vi "Test Tag For New Test Method Correct When dot in Test name.vi"(8 "error in (no error)":errorcluster, 11 "Result Model Tests in":refnum<class "Result Model Test Enumeration.lvclass">) -> (0 "error out":errorcluster, 3 "Result Model Tests out":refnum<class "Result Model Test Enumeration.lvclass">)   [LabVIEW 2020, in "Result Model Test Enumeration.lvclass"]
uses:
  Result Model Test Enumeration.lvclass
  source/User Interface/Result Model/Result Model.lvclass
  206db1ee-aa99-40b9-8881-171f2a77c34b.vi
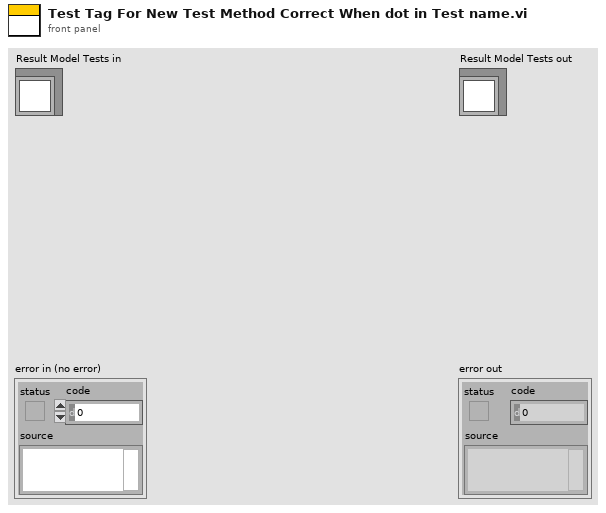
[diagram p1: front panel]
types:
  T1 = cluster{"Left Cell String":string, "Child Text":string[], "Child Tag":string, "Item Indent":i32, "Child Only?":bool, "Glyph Index":i32}[]
  T2 = cluster{"Left Cell String":string, "Child Text":string[], "Child Tag":string, "Item Indent":i32, "Child Only?":bool, "Glyph Index":i32}
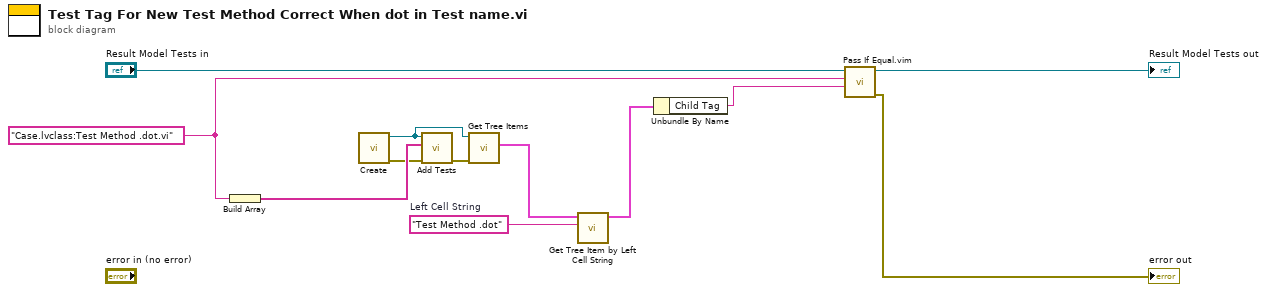
[diagram p0: block diagram]
diagram:
  w5 = "Case.lvclass:Test Method .dot.vi" ("String")
  w10 = "Test Method .dot"  # Left Cell String
  n1 = Build Array(w5) -> (w6:string[])
  n2 = call "Create.vi"() -> ("error out"=w3:errorcluster, "Result Model out"=w1:refnum<class "Result Model.lvclass">)  [unwired: 10 in]
  n3 = call "Add Tests.vi"("error in (no error)"=w3, "Tests"=w6, "Result Model by Reference In"=w1) -> ("error out"=w2:errorcluster)  [unwired: 8 in]
  n4 = call "Get Tree Items.vi"("error in (no error)"=w2, "Result Model by Reference In"=w1) -> ("Tree Items"=w11:T1)  [unwired: 8 in, 1 out]
  n5 = call "Get Tree Item by Left Cell String.vi"("Left Cell String"=w10, "Tree Items"=w11) -> ("Item"=w8:T2)  [unwired: 9 in]
  n6 = Unbundle By Name(w8) -> ("Child Tag"=w7:string)
  n7 = call "Pass If Equal.vim"("Actual"=w7, "Expected"=w5, "LUnit Test Case In"="Result Model Tests in") -> ("error out"=→"error out":errorcluster, "LUnit Test Case Out"=→"Result Model Tests out":refnum<class "Result Model Test Enumeration.lvclass">)  [unwired: 7 in]
